vi "sub vi3.vi"(2 "Numeric 4":dbl, 3 "Numeric 3":dbl) -> (0 "Numeric 2":dbl, 1 "Numeric":dbl)   [LabVIEW 2023]
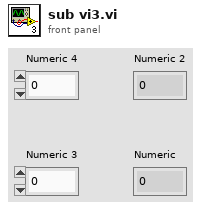
[diagram p1: front panel]
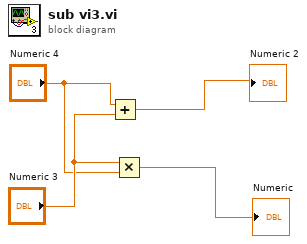
[diagram p0: block diagram]
diagram:
  n1 = Add(x="Numeric 4", y="Numeric 3") -> (x+y=→"Numeric 2":dbl)
  n2 = Multiply(x="Numeric 3", y="Numeric 4") -> (x*y=→"Numeric":dbl)
